vi "inference.vi"() -> ()   [LabVIEW 2024]
uses:
  <vilib>/Python/Open Anaconda Python Session.vi
panel:
  out "inference_path":path
  out "image_path":string
  out "return value":string
  out "string":string
  out "Application Directory":path
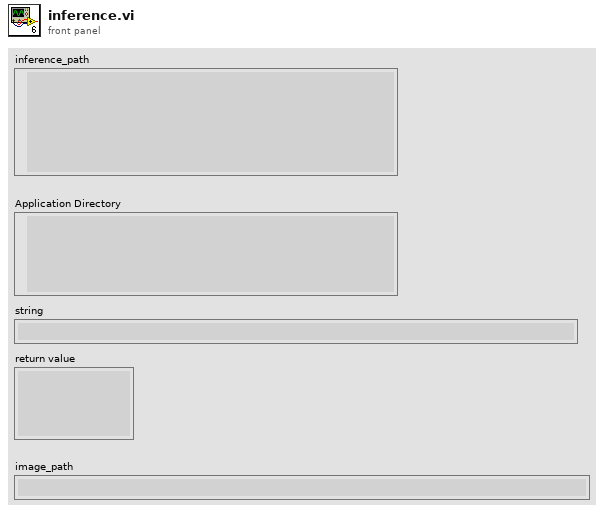
[diagram p1: front panel]
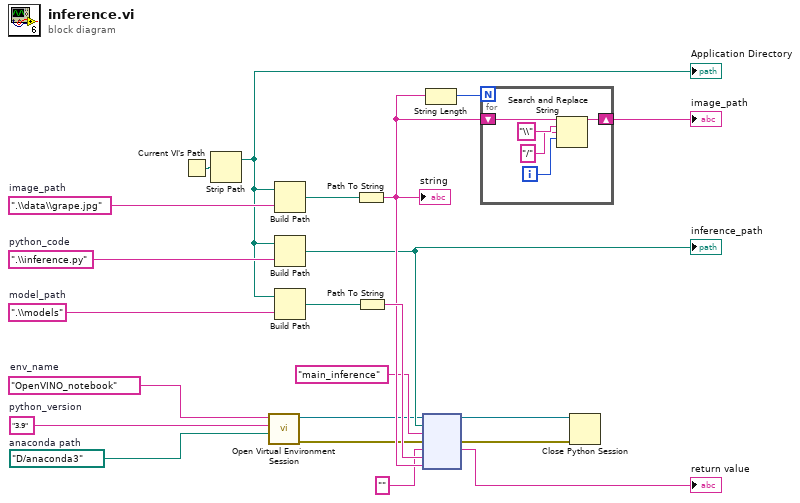
[diagram p0: block diagram]
diagram:
  w6 = path "D:/anaconda3"  # anaconda path
  w7 = "OpenVINO_notebook"  # env_name
  w8 = "3.9"  # python_version
  w14 = ".\\inference.py"  # python_code
  w20 = ".\\models"  # model_path
  w22 = ".\\data\\grape.jpg"  # image_path
  n1 = Current VI's Path() -> (path=w2:path)
  n2 = Strip Path(path=w2) -> (stripped path=w1:path)  [unwired: 1 out]
  "Application Directory" <- w1
  n3 = call-poly <vilib>:"Open Virtual Environment Session.vi"("Anaconda path"=w6, "Python version"=w8, "Env name"=w7) -> ("error out"=w4:errorcluster, "session out"=w5:refnum<k35>)  [unwired: 7 in]
  n4 = Build Path(base path=w1, name or relative path=w22) -> (appended path=w21:path)
  n5 = Build Path(base path=w1, name or relative path=w14) -> (appended path=w13:path)
  "inference_path" <- w13
  n6 = Build Path(base path=w1, name or relative path=w20) -> (appended path=w19:path)
  n7 = Path To String(path=w21) -> (string=w16:string)
  "string" <- w16
  n8 = Path To String(path=w19) -> (string=w18:string)
  n9 = node(w5, w13, "main_inference" ("function name"), w4, "", w18, w16) -> (w12:refnum<k35>, w11:errorcluster, →"return value":string)  [unwired: 2 in, 2 out]
  n10 = String Length(string=w16) -> (length=w17:i32)
  n11 = for {
    N: w17 -> [_]
    shift-right: [w23] -> w15
    shift-left: w16 -> [w26]
    i -> [w24]
    n12 = Search and Replace String(input string=w26, search string="\\", replace string="/" ("replace string (\"\")"), offset=w24) -> (result string=w23:string)  [unwired: 4 in, 3 out]
  }
  "image_path" <- w15
  n13 = Close Python Session(session in=w12, error in=w11) -> ()  [unwired: 1 out]
